vi "Move Subpanel.vi"(4 "Visible (True)":bool=TRUE, 6 "Loop Number (16)":i32=16, 8 "error in (no error)":errorcluster, 9 "Insertion Request Time":timestamp, 10 "Position":T1, 11 "Protected Subpanel":T2) -> (0 "error out":errorcluster, 3 "Protected Subpanel":T2)   [LabVIEW 2020, in "IViewable.lvlib" / "ProtectedSubpanel.lvclass"]
uses:
  <vilib>/gpm_packages/@cs/mva-viewable/Source/IViewable/ProtectedSubpanel/ProtectedSubpanel.lvclass
  <vilib>/gpm_packages/@cs/mva-viewable/Source/IViewable/ProtectedSubpanel/Protected Subpanel Reference.ctl
  <vilib>/Utility/miscctls.llb/LVPositionTypeDef.ctl
  <vilib>/gpm_packages/@cs/mva-viewable/Source/IViewable/ProtectedSubpanel/ProtectedSubpanel.lvclass/ProtectedSubpanel.ctl
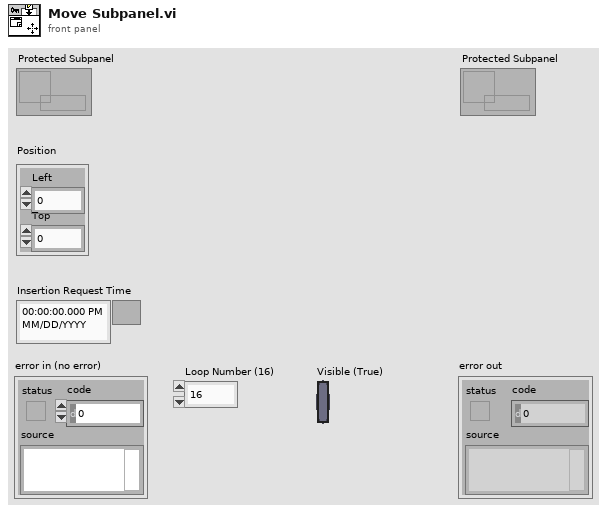
[diagram p1: front panel]
types:
  T1 = typedef "LVPositionTypeDef.ctl" = cluster{"Left":i32, "Top":i32}
  T2 = typedef "IViewable.lvlib/ProtectedSubpanel.lvclass/Protected Subpanel Reference.ctl" = refnum<data-value>
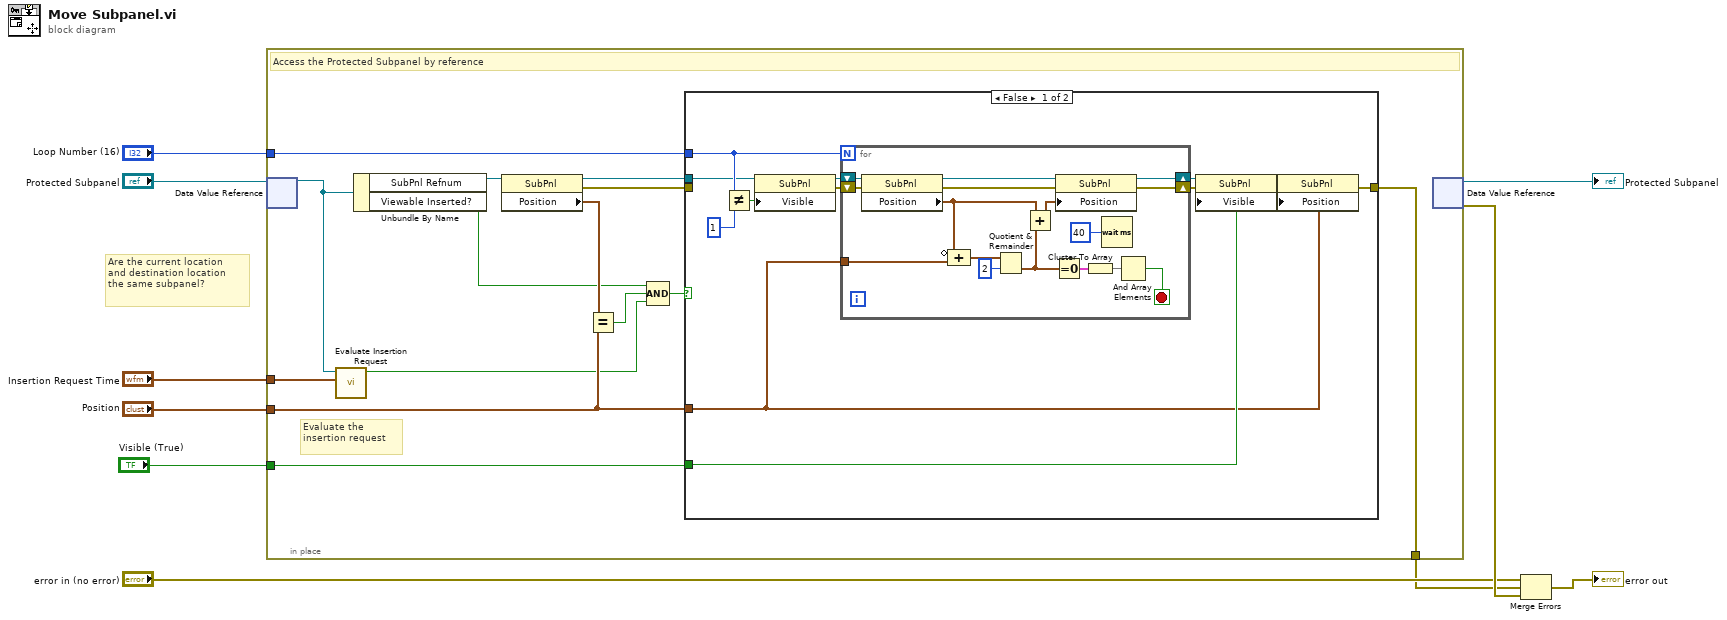
[diagram p0: block diagram]
diagram:
  # "Are the current location\nand destination location\nthe same subpanel?"
  n1 = in-place {
    in-place-border: "Insertion Request Time" -> [w24]
    in-place-border: "Position" -> [w19]
    in-place-border: "Loop Number (16)" -> [w20]
    in-place-border: "Visible (True)" -> [w18]
    in-place-border: [w15] -> w1
    # "Evaluate the\ninsertion request"
    # "Access the Protected Subpanel by reference"
    n2 = in-place-dvr #1("Protected Subpanel") -> (w23:refnum<class "ProtectedSubpanel.lvclass">)  [unwired: 1 out]
    n3 = call <vilib>:"Evaluate Insertion Request.vi"("Insertion Request Time"=w24, "ProtectedSubpanel"=w23) -> ("Perform Insertion?"=w13:bool)  [unwired: 9 in]
    n4 = Unbundle By Name(w23) -> ("SubPnl Refnum"=w21:refnum<vi>, "Viewable Inserted?"=w11:bool)
    n5 = property class="SubPnl"(reference=w21) -> (reference out=w16:refnum<vi>, error out=w17:errorcluster, "Position"=w22:T1)  [unwired: 1 in]
    n6 = Equal?(x=w22, y=w19) -> (x = y?=w14:bool)
    n7 = Compound Arithmetic op=AND(w11, w14, w13) -> (w12:bool)
    n8 = case shown="False" w12 {
      tunnel: [w36 w54] -> w15
      tunnel: w20 -> [w33 _]
      tunnel: w18 -> [w27 _]
      tunnel: w16 -> [w26 _]
      tunnel: w19 -> [w25 _]
      tunnel: w17 -> [_ w54]
      frame False {
        n9 = Not Equal?(x=w33, y=1) -> (x != y?=w31:bool)
        n10 = property class="SubPnl"(reference=w26, "Visible"=w31) -> (reference out=w34:refnum<vi>, error out=w35:errorcluster)  [unwired: 1 in]
        n11 = for {
          N: w33 -> [_]
          shift-right: [w51] -> w29
          shift-left: w34 -> [w53]
          shift-right: [w44] -> w37
          shift-left: w35 -> [w52]
          tunnel: w25 -> [w38]
          stop <- w40 stop-if-true
          n12 = property class="SubPnl"(reference=w53, error in=w52) -> (reference out=w49:refnum<vi>, error out=w50:errorcluster, "Position"=w41:T1)
          n13 = Compound Arithmetic op=ADD(invert w41, w38) -> (w47:T1)
          n14 = Quotient & Remainder(x=w47, y=2) -> (floor(x/y)=w45:T1)  [unwired: 1 out]
          n15 = Add(x=w41, y=w45) -> (x+y=w48:T1)
          n16 = Equal To 0?(x=w45) -> (x = 0?=w43:cluster{"Left":bool, "Top":bool})
          n17 = property class="SubPnl"(reference=w49, error in=w50, "Position"=w48) -> (reference out=w51:refnum<vi>, error out=w44:errorcluster)
          n18 = Cluster To Array(cluster=w43) -> (array=w39:bool[])
          n19 = Wait (ms)(milliseconds to wait=u32 40) -> ()  [unwired: 1 out]
          n20 = And Array Elements(Boolean array=w39) -> (logical AND=w40:bool)
        }
        n21 = property class="SubPnl"(reference=w29, error in=w37, "Visible"=w27) -> (reference out=w28:refnum<vi>, error out=w30:errorcluster)
        n22 = property class="SubPnl"(reference=w28, error in=w30, "Position"=w25) -> (error out=w36:errorcluster)  [unwired: 1 out]
      }
      frame True {
      }
    }
    n23 = in-place-dvr #1() -> (→"Protected Subpanel":T2, w7:errorcluster)  [unwired: 1 in]
  }
  n24 = Merge Errors("error in (no error)", w1, w7) -> (→"error out":errorcluster)
